vi "onPostSuiteSlippage.vi"(7 "TraceabilityMatrix in":refnum<class "TraceabilityMatrix.lvclass">, 11 "Leaf.TestSuite":refnum<class "Leaf.TestSuite.lvclass">) -> (0 "error out":errorcluster, 3 "Leaf.TestSuite":refnum<class "Leaf.TestSuite.lvclass">)   [LabVIEW 2021, in "Bananas.lvlib" / "TraceabilityMatrix.lvclass"]
uses:
  TraceabilityMatrix.lvclass
  Leaf.TestSuite/Leaf.TestSuite.lvclass
  C:/Repositories/LVOS/Bananas/lv-src/Bananas/Leaf/Leaf.lvclass
  TraceabilityMatrix.lvclass/TraceabilityMatrix.ctl
  Leaf/Leaf.lvclass
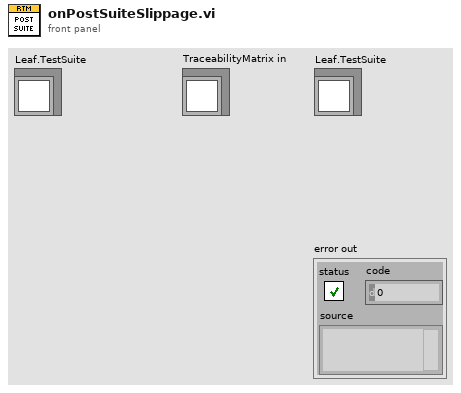
[diagram p1: front panel]
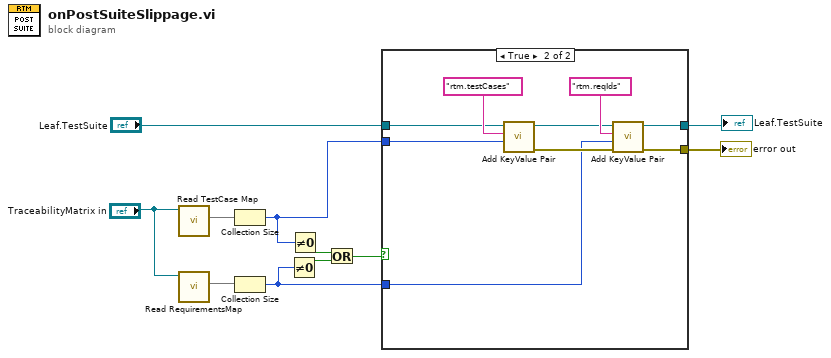
[diagram p0: block diagram]
diagram:
  n1 = call "Read TestCase Map.vi"("TraceabilityMatrix in"="TraceabilityMatrix in") -> ("TestCaseMap"=w11:map{string, set{string}})  [unwired: 9 in, 1 out]
  n2 = call "Read RequirementsMap.vi"("TraceabilityMatrix in"="TraceabilityMatrix in") -> ("RequirementMap"=w10:map{string, set{string}})  [unwired: 9 in, 1 out]
  n3 = Collection Size(1:w11) -> (0:w9:i32)
  n4 = Collection Size(1:w10) -> (0:w8:i32)
  n5 = Not Equal To 0?(x=w8) -> (x != 0?=w6:bool)
  n6 = Not Equal To 0?(x=w9) -> (x != 0?=w7:bool)
  n7 = Or(x=w7, y=w6) -> (x .or. y?=w5:bool)
  n8 = case shown="True" w5 {
    tunnel: "Leaf.TestSuite" -> [w12 w20]
    tunnel: [w12 w17] -> w3
    tunnel: [_ w15] -> w2
    tunnel: w9 -> [_ w14]
    tunnel: w8 -> [_ w13]
    frame False {
    }
    frame True {
      n9 = call "Add KeyValue Pair.vi"("value"=w14, "key"="rtm.testCases", "Leaf in"=w20) -> ("error out"=w16:errorcluster, "Leaf out"=w18:refnum<class "Leaf.TestSuite.lvclass">)  [unwired: 7 in]
      n10 = call "Add KeyValue Pair.vi"("error in (no error)"=w16, "value"=w13, "key"="rtm.reqIds", "Leaf in"=w18) -> ("error out"=w15:errorcluster, "Leaf out"=w17:refnum<class "Leaf.TestSuite.lvclass">)  [unwired: 6 in]
    }
  }
  "error out" <- w2
  "Leaf.TestSuite" <- w3
